vi "PCAN.vi"(8 "error in (no error)":errorcluster, 10 "DUT":string) -> (0 "error in (out)":errorcluster)   [LabVIEW 2024, in "PCANusb_DTU.lvlib"]
doc: "This template is for the Queued Message Handler design pattern.\n\nThe Event Handling Loop generates messages based on user interface actions.\n\nThe Message Handling Loop processes messages generated by the Event Handling Loop, or by other messages. The messages are string values, so new messages can be added easily to the Message Cases case structure in the Message Handling Loop. Each message cluster can also provide an optional value for Message Data, which is a variant that can be converted to whatever message-specific data is required."
uses:
  PCANusb_DTU.lvlib
  support/CAN_MSGs.ctl
  support/CAN_Frames_ctrl.ctl
  support/Framing datas.ctl
  <vilib>/xnet/xnet.llb/XNET Frame CAN.ctl
  <vilib>/xnet/xnet.llb/XNET Frame Type CAN.ctl
  controls/PCAN UI Data.ctl
  support/CAN_Read.ctl
  PrivateControls/FGV_Queue_Control.ctl
  support/PCAN_Global.vi
  Launcher/SubVI/Global 1.vi
  support/Write_frames.vi
  <vilib>/Utility/error.llb/Error Cluster From Error Code.vi
  <vilib>/ErrorRing/Error Ring.xnode
  support/Message Queue/PCAN Message Queue.lvlib
  support/User Event - Stop/PCAN User Event - Stop.lvlib
  <userlib>/PCANBasic/PCANBasic.lvlib
  Launcher/Launcher_DTU.lvlib
  <vilib>/xnet/xnet.llb/XNET Convert (Signal to Frame CAN).vi
panel:
  in  "Config":string
  out "Barcode data":u8[][](array[numeric]) format="%.0x"
  out "CAN_Frames.CAN_ID":u32 format="%.0x"
  out "function return":u32
  out "Channel":u16 format="%.0x"
  out "TPCANMsg":T1[](array[typedef]) {"payload" format="%x"; "timestamp" format="%<%.7X\n%x>T"; "type" items=["CAN Data"=0, "CAN Remote"=1, "CAN Bus Error"=2, "CAN 2.0 Data"=8, "CAN FD Data"=16, "CAN FD+BRS Data"=24, "J1939 Data"=192, "Delay"=224, "Log Trigger"=225, "Start Trigger"=226]; "identifier" format="%x"}
  out "frame data":T1[](array[typedef]) {"payload" format="%x"; "timestamp" format="%<%.7X\n%x>T"; "type" items=["CAN Data"=0, "CAN Remote"=1, "CAN Bus Error"=2, "CAN 2.0 Data"=8, "CAN FD Data"=16, "CAN FD+BRS Data"=24, "J1939 Data"=192, "Delay"=224, "Log Trigger"=225, "Start Trigger"=226]; "identifier" format="%x"}
  out "CAN_bit frame":bool[][](array[boolean])
  in  "CAN_MSGs":T3={"Scaling Factor"=1, "Physical value"=0.0, "CAN_Frames"={"CAN_ID"=0, "MSGTYPE"=128, "Payload"=[], "Length"=0}, "Offset value"=0.0, "Framing datas"=[], "CAN_Frame Enable"=FALSE, "Add Signal"=FALSE, "Delete Signal"=FALSE, "Signal Values"=[], "Time(ms)"=0.0, "Repetition"=FALSE, "Delay"=FALSE, "Delay time"=0.0} {"CAN_Frames"."Payload" format="%.0x"; "CAN_Frames"."MSGTYPE" items=["STATUS"=128, "EXTENDED"=2, "RTR"=1, "DATA MSG"=0]; "CAN_Frames"."CAN_ID" format="%.0x"}
  out "queue name":string
  out "Display <Replace Me>":string
  in  "Read_PCAN":bool
  in  "Write_PCAN":bool
  in  "Exit":bool
  # "Need to build a logic which takes all the bit information,\nbyte info ,Starting bit , Bit length, for each signal with add button to add\nmuch signals manually. And also an option to write payload data for the \nsetup.  - Done."
  # "0     1     2     3     4     5     6     7"
  # "0"
  # "1"
  # "2"
  # "3"
  # "4"
  # "5"
  # "6"
  # "7"
  # "0     1     2     3     4     5     6     7"
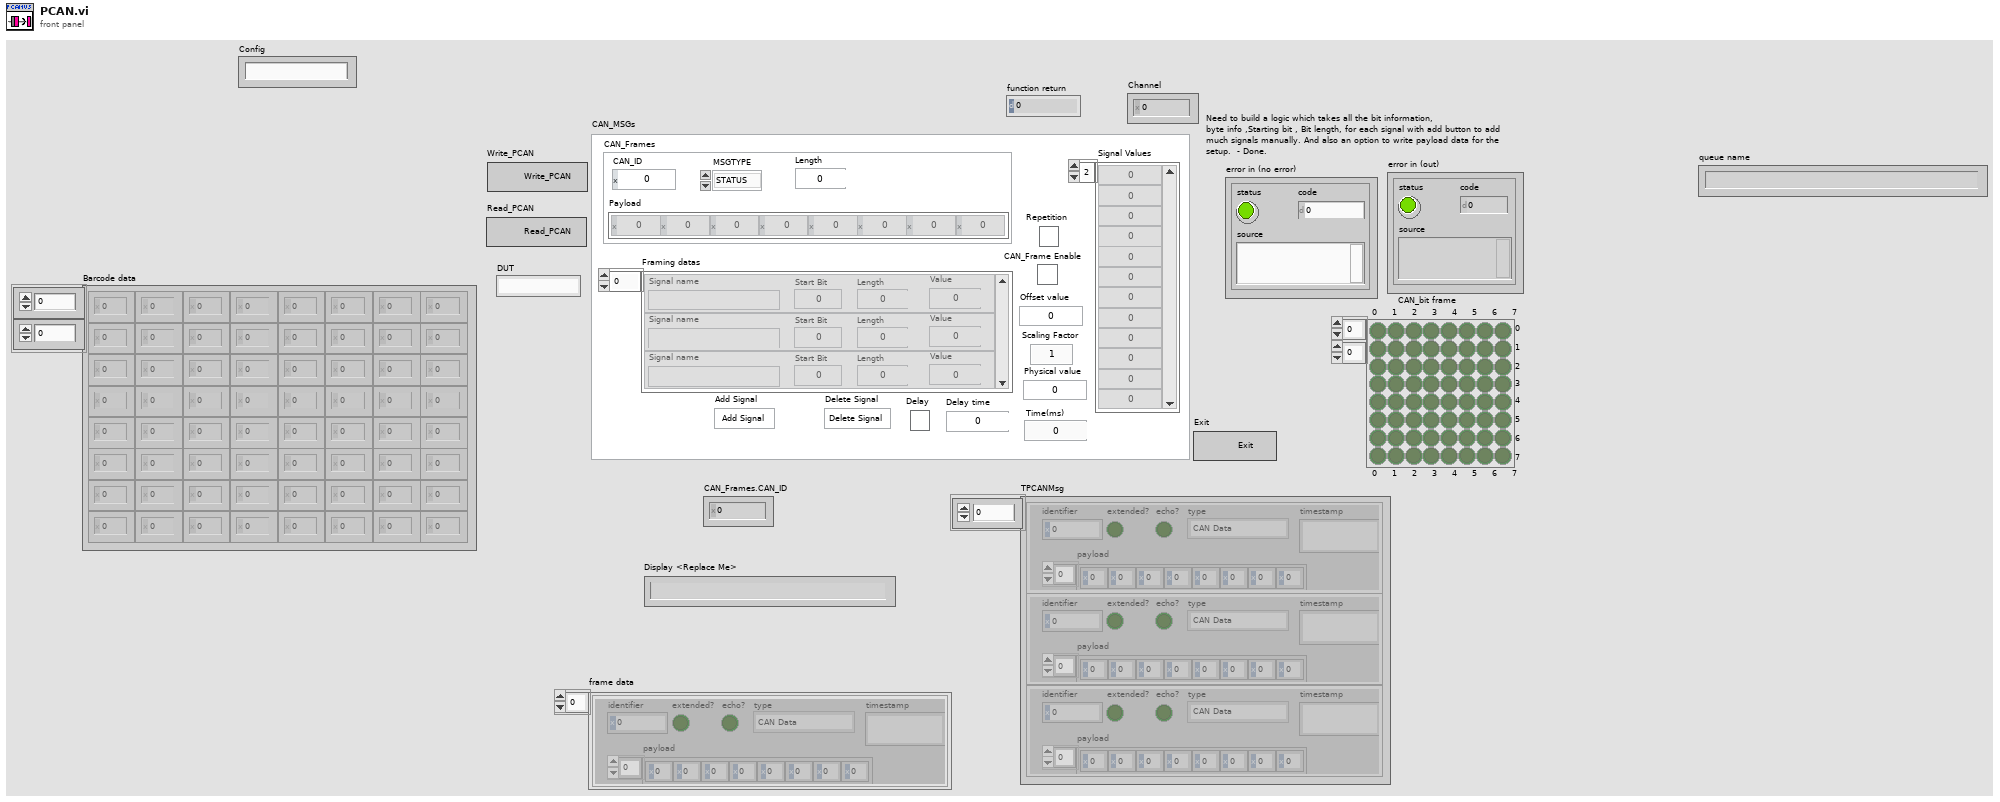
[diagram p1: front panel]
types:
  T1 = typedef "XNET Frame CAN.ctl" = cluster{"timestamp":timestamp, "payload":u8[], "identifier":u32, "type":T2, "extended?":bool, "echo?":bool}
  T2 = typedef "XNET Frame Type CAN.ctl" = u8
  T3 = typedef "PCANusb_DTU.lvlib/CAN_MSGs.ctl" = cluster{"Scaling Factor":u16, "Physical value":dbl, "CAN_Frames":T4, "Offset value":dbl, "Framing datas":T5[], "CAN_Frame Enable":bool, "Add Signal":bool, "Delete Signal":bool, "Signal Values":dbl[], "Time(ms)":dbl, "Repetition":bool, "Delay":bool, "Delay time":dbl}
  T4 = typedef "PCANusb_DTU.lvlib/CAN_Frames_ctrl.ctl" = cluster{"CAN_ID":u32, "MSGTYPE":u8, "Payload":u8[], "Length":u8}
  T5 = typedef "PCANusb_DTU.lvlib/Framing datas.ctl" = cluster{"Signal name":string, "Start Bit":u8, "Length":u8, "Value":u16}
  T6 = cluster{"Message":string, "Message Data":variant}
  T7 = typedef "PCANusb_DTU.lvlib/PCAN UI Data.ctl" = cluster{"DLL_Path":path, "DLL_Path 2":path, "DUT":i32, "CAN_MSGs_Write":T3, "CAN_Array":T3[], "TPCANMsg":cluster{"timestamp":timestamp, "payload":u8[], "identifier":u32, "type":T2, "extended?":bool, "echo?":bool}[], "CAN_Read":T8, "notifier out":refnum<notifier>, "TPCANMsg 2":cluster{"timestamp":timestamp, "payload":u8[], "identifier":u32, "type":T2, "extended?":bool, "echo?":bool}[], "Channel":u16, "reference":refnum<vi>[], "CANand ref":u32[], "CANID Found":bool, "Serial no.":u8[][], "Repeatno.":u8, "GPS":u8[][], "imei":u8[][], "iccid":u8[][], "macid":u8[], "P_queue":refnum<queue>, "Config":string}
  T8 = typedef "PCANusb_DTU.lvlib/CAN_Read.ctl" = cluster{"Database":refnum<k21>, "Signal":refnum<k21>, "BYTES":u32[], "ReadPayload":u8[], "String_Data":string, "ReadValue":dbl, "CANID":u32, "SERVICE ID":u32, "SUB-SERVICE ID":u32, "DELAY ":bool, "Delay time(ms)":dbl}
  T9 = typedef "PCANusb_DTU.lvlib/PCAN Message Queue.lvlib/All Message Queues.ctl" = cluster{"UI":refnum<queue>, "QSM":refnum<queue>}
  T10 = cluster{"timestamp":timestamp, "payload":u8[], "identifier":u32, "type":T2, "extended?":bool, "echo?":bool}[]
  T11 = typedef "PCANusb_DTU.lvlib/FGV_Queue_Control.ctl" = enum16{"Release", "Flush", "Get", "Set"}
  T12 = enum16{"Read", "Write", "All_sections", "All_values", "Remove key&section"}
  T13 = cluster{"millis":u32, "millis_overflow":u16, "micros":u16}
  T14 = cluster{"ID":u32, "MSGTYPE":u8, "LEN":u8, "DATA[0]":u8, "DATA[1]":u8, "DATA[2]":u8, "DATA[3]":u8, "DATA[4]":u8, "DATA[5]":u8, "DATA[6]":u8, "DATA[7]":u8}
  T15 = cluster{"timestamp":timestamp, "payload":u8[], "identifier":u32, "type":T2, "extended?":bool, "echo?":bool}
  T16 = cluster{"ID":u32, "MSGTYPE":u8, "LEN":u8, "aDATA":u8[]}
  T17 = typedef "PCAN_ERROR.ctl" = i32
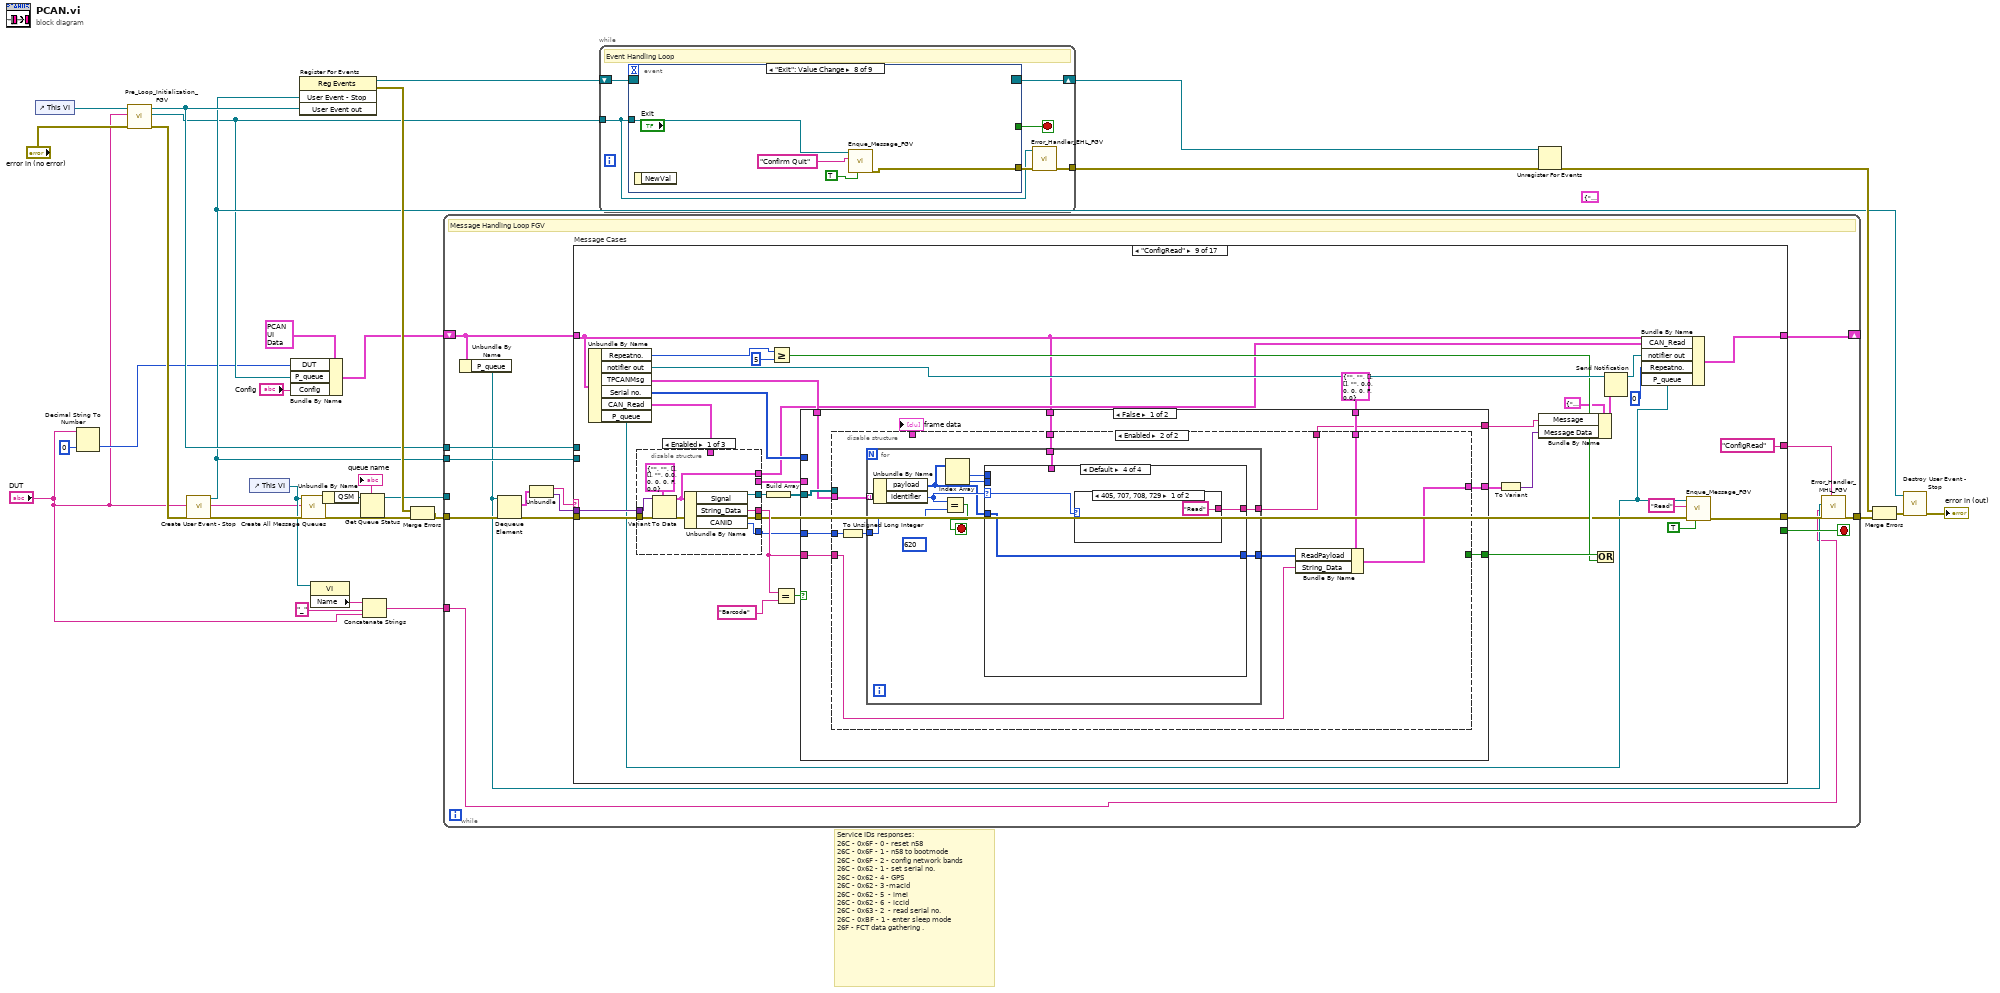
[diagram p0: block diagram]
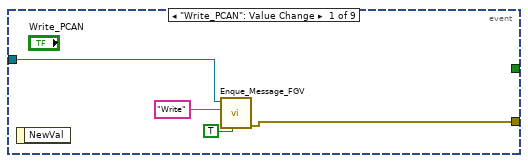
[diagram p2: hidden frame]
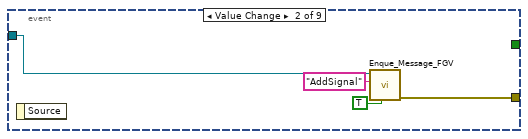
[diagram p3: hidden frame]
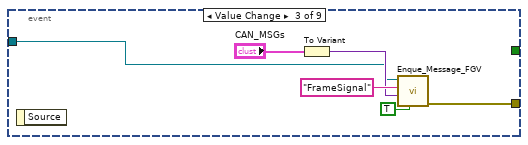
[diagram p4: hidden frame]
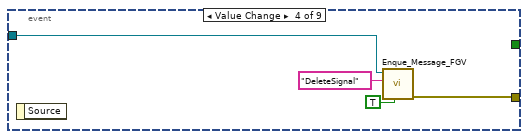
[diagram p5: hidden frame]
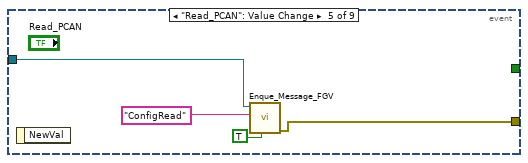
[diagram p6: hidden frame]
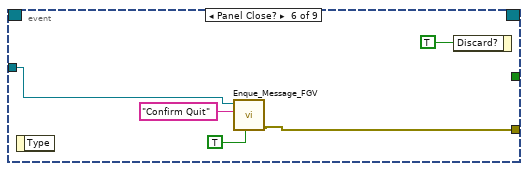
[diagram p7: hidden frame]
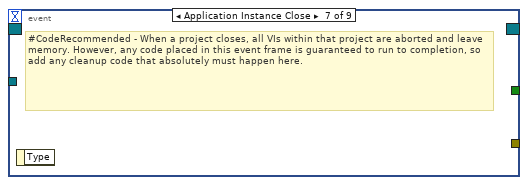
[diagram p8: hidden frame]
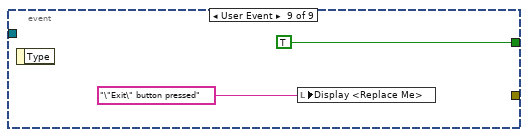
[diagram p9: hidden frame]
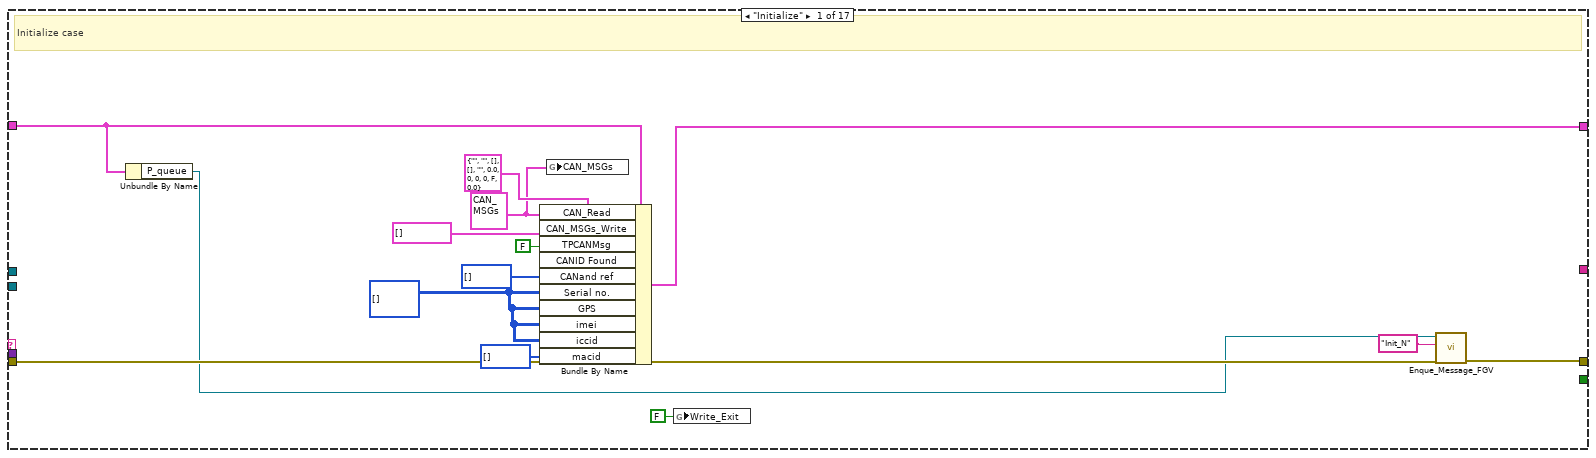
[diagram p10: hidden frame]
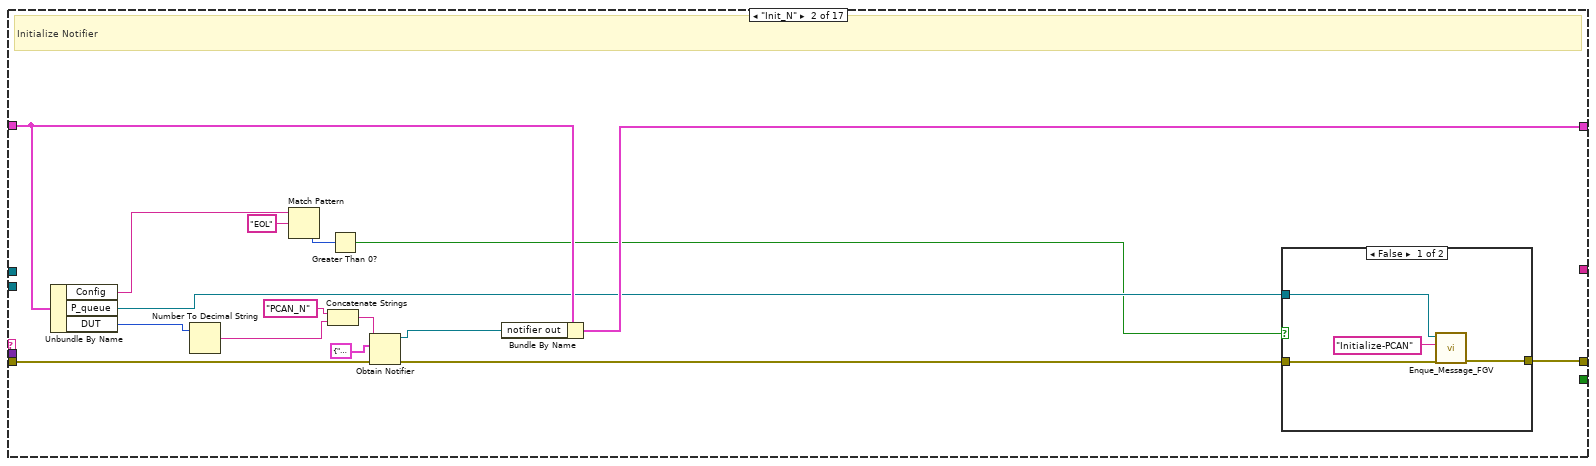
[diagram p11: hidden frame]
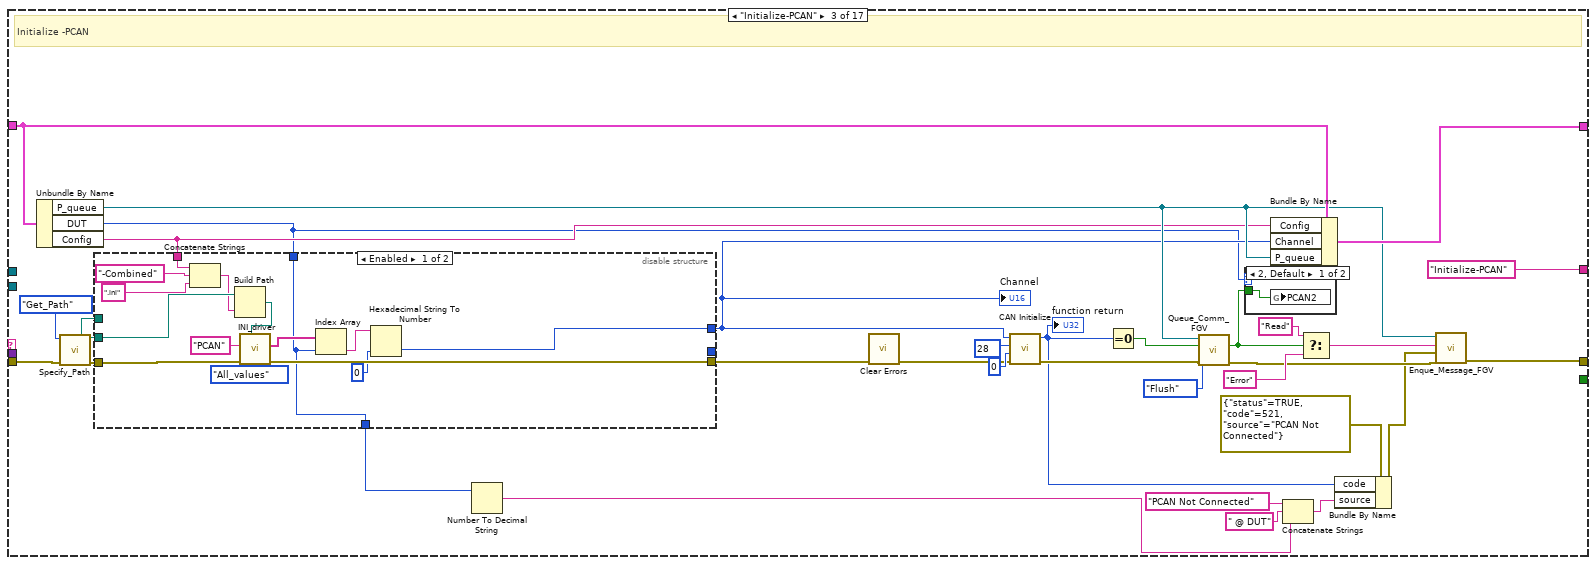
[diagram p13: hidden frame]
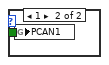
[diagram p14: hidden frame]
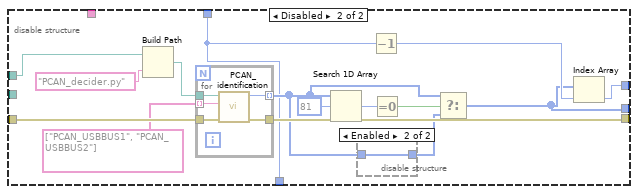
[diagram p15: hidden frame]
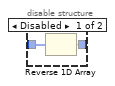
[diagram p16: hidden frame]
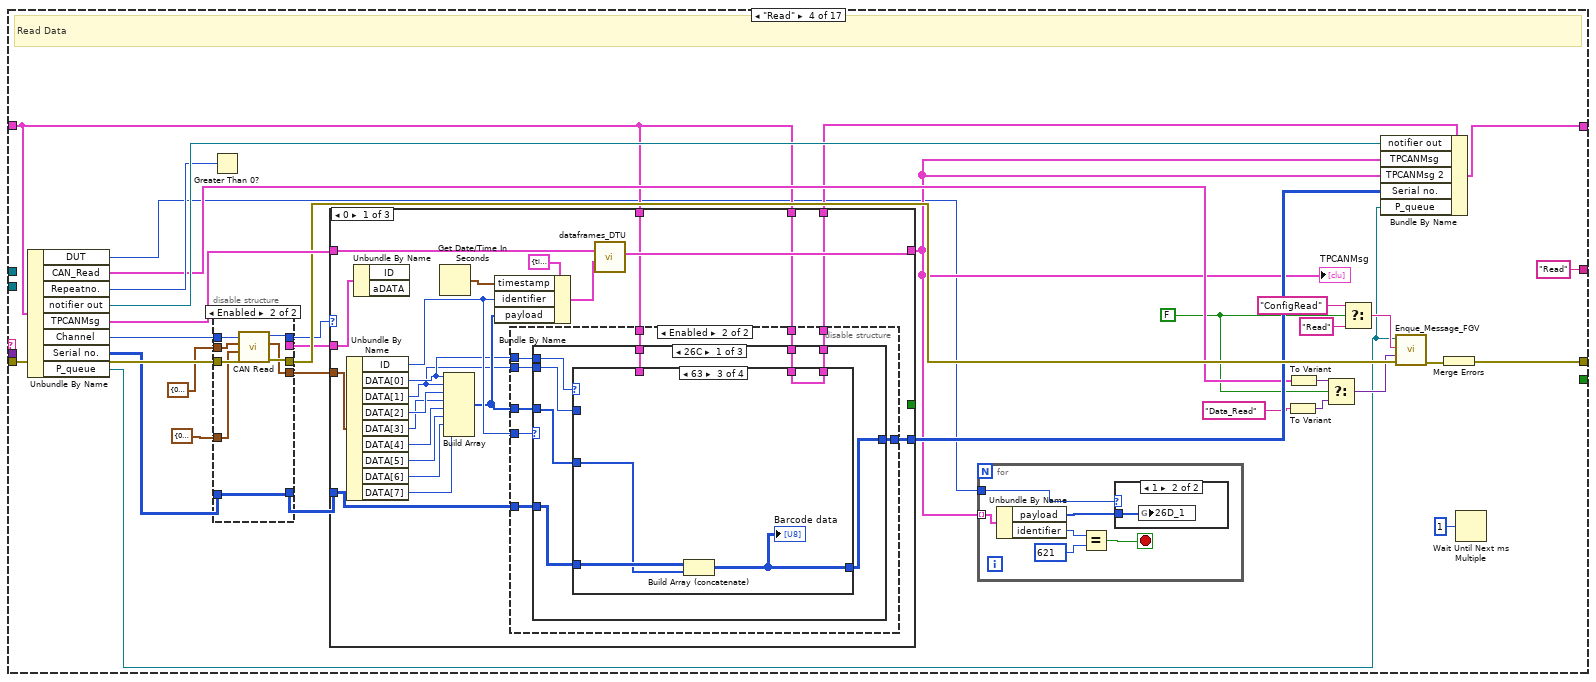
[diagram p17: hidden frame]
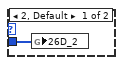
[diagram p18: hidden frame]
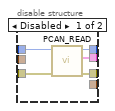
[diagram p19: hidden frame]
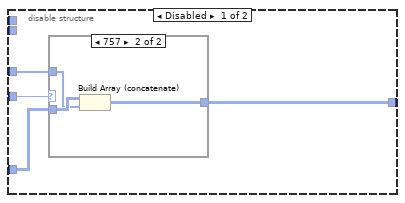
[diagram p20: hidden frame]
diagram:
  (unwired) T6 {"Message"="", "Message Data"=variant} ("notification")
  # "Service IDs responses: \n26C - 0x6F - 0 - reset n58\n26C - 0x6F - 1 - n58 to bootmode\n26C - 0x6F - 2 - config network bands\n26C - 0x62 - 1 - set serial no.\n26C - 0x62 - 4 - GPS\n26C - 0x62 - 3 -macid\n26C - 0x62 - 5  - imei\n26C - 0x62 - 6  - iccid\n26C - 0x63 - 2  - read serial no.\n26C - 0xBF - 1 - enter sleep mode\n26F - FCT data gathering ."
  n1 = control-ref of="This VI"() -> (w19:refnum<vi>)
  n2 = Decimal String To Number(string="DUT", default (0L)=0 ("default (0 I32)")) -> (number=w6:i32)  [unwired: 1 in, 1 out]
  n3 = call "Pre_Loop_Initialization_FGV.vi"("error in (no error)"="error in (no error)", "DUT"="DUT", "VI in"=w19) -> ("error out"=w17:errorcluster, "queue out"=w9:refnum<queue>, "User Event out"=w12:refnum<user-event>)  [unwired: 6 in]
  n4 = call "Create User Event - Stop.vi"("error in (no error)"=w17) -> ("error out"=w13:errorcluster, "User Event - Stop"=w11:refnum<user-event>)  [unwired: 9 in]
  n5 = control-ref of="This VI"() -> (w5:refnum<vi>)
  n6 = Bundle By Name(cluster=T7 {"DLL_Path"=path "", "DLL_Path 2"=path "", "DUT"=1, "CAN_MSGs_Write"={"Scaling Factor"=0, "Physical value"=128.0, "CAN_Frames"={"CAN_ID"=0, "MSGTYPE"=128, "Payload"=[], "Length"=0}, "Offset value"=0.0, "Framing datas"=[], "CAN_Frame Enable"=FALSE, "Add Signal"=FALSE, "Delete Signal"=FALSE, "Signal Values"=[], "Time(ms)"=0.0, "Repetition"=FALSE, "Delay"=FALSE, "Delay time"=0.0}, "CAN_Array"=[], "TPCANMsg"=[{"timestamp"=timestamp(0 s since 1904-01-01), "payload"=[], "identifier"=0, "type"=0, "extended?"=FALSE, "echo?"=FALSE}, {"timestamp"=timestamp(0 s since 1904-01-01), "payload"=[], "identifier"=0, "type"=0, "extended?"=FALSE, "echo?"=FALSE}], "CAN_Read"={"Database"="", "Signal"="", "BYTES"=[], "ReadPayload"=[], "String_Data"="", "ReadValue"=0.0, "CANID"=0, "SERVICE ID"=0, "SUB-SERVICE ID"=0, "DELAY "=FALSE, "Delay time(ms)"=0.0}, "notifier out"=refnum, "TPCANMsg 2"=[{"timestamp"=timestamp(0 s since 1904-01-01), "payload"=[], "identifier"=0, "type"=0, "extended?"=FALSE, "echo?"=FALSE}, {"timestamp"=timestamp(0 s since 1904-01-01), "payload"=[], "identifier"=0, "type"=0, "extended?"=FALSE, "echo?"=FALSE}], "Channel"=81, "reference"=[], "CANand ref"=[], "CANID Found"=FALSE, "Serial no."=[], "Repeatno."=0, "GPS"=[], "imei"=[], "iccid"=[], "macid"=[], "P_queue"=refnum, "Config"=""} ("Data Cluster"), "DUT"=w6, "P_queue"=w9, "Config"="Config") -> (w10:T7)
  n7 = register-events(w11, w12) -> (reference out=w22:refnum<event-registration>, error out=w20:errorcluster)  [unwired: 2 in]
  n8 = call "Create All Message Queues.vi"("error in (no error)"=w13, "DUT"="DUT", "This VI"=w5) -> ("error out"=w31:errorcluster, "Message Queues out"=w30:T9)  [unwired: 7 in]
  n9 = property class="VI"(reference=w5) -> ("Name"=w4:string)  [unwired: 1 in, 2 out]
  n10 = Unbundle By Name(w30) -> ("QSM"=w28:refnum<queue>)
  n11 = Get Queue Status(queue=w28) -> (queue out=w15:refnum<queue>, queue name=→"queue name":string)  [unwired: 2 in, 6 out]
  n12 = Concatenate Strings(w4, "_" ("string"), "DUT") -> (w1:string)
  n13 = Merge Errors(w20, w31) -> (w21:errorcluster)
  n14 = while {
    tunnel: w15 -> [_]
    shift-right: [w46] -> _
    shift-left: w10 -> [w38]
    tunnel: w12 -> [w44]
    tunnel: w21 -> [w43]
    tunnel: [w40] -> w29
    tunnel: w11 -> [w39]
    tunnel: w1 -> [w33]
    stop <- w45 stop-if-true
    # "Message Handling Loop FGV"
    n15 = Unbundle By Name(w38) -> ("P_queue"=w34:refnum<queue>)
    n16 = Dequeue Element(queue=w34, error in (no error)=w43) -> (element=w37:T6, error out=w42:errorcluster)  [unwired: 1 in, 2 out]
    n17 = Unbundle(w37) -> ("Message"=w36:string, "Message Data"=w35:variant)
    n18 = case "Message Cases" shown="\"ConfigRead\"" w36 {
      selector: w36 -> [_ _ _ _ _ _ _ _ _ _ _ _ _ _ _ _ w624]
      tunnel: w42 -> [w58 w75 w102 w184 w314 w364 w374 w387 w424 w558 w567 w577 w582 w590 w599 w609 _]
      tunnel: [w60 w76 w113 w186 w325 w358 w371 w383 w397 w557 w566 w578 w579 w585 w606 w608 w623] -> w41
      tunnel: w38 -> [w48 w73 w97 w160 w329 w356 w367 w382 w396 w556 w565 w572 w583 w584 w602 w614 w625]
      tunnel: [w57 w68 w112 w181 w326 w357 w370 w385 w421 w554 w563 w572 w583 w584 w602 w614 w625] -> w46
      tunnel: [_ _ _ _ _ _ _ _ _ _ _ _ _ _ _ TRUE _] -> w45
      tunnel: w35 -> [_ _ _ _ _ w363 _ w386 w423 _ _ w576 _ w589 _ _ _]
      tunnel: w44 -> [_ _ _ _ _ _ _ _ _ _ _ _ _ _ _ w620 _]
      tunnel: w39 -> [_ _ _ _ _ _ _ _ _ _ _ _ _ _ _ w617 _]
      tunnel: [_ _ "Initialize-PCAN" ("Case") "Read" ("Case") "Write" ("Case") _ _ _ "ConfigRead" ("Case") _ _ _ _ _ _ _ _] -> w32
      frame "Initialize" {
        w50 = u8[][] [] ("Payload")
        w51 = T3 {"Scaling Factor"=1, "Physical value"=0.0, "CAN_Frames"={"CAN_ID"=0, "MSGTYPE"=128, "Payload"=[], "Length"=0}, "Offset value"=0.0, "Framing datas"=[], "CAN_Frame Enable"=FALSE, "Add Signal"=FALSE, "Delete Signal"=FALSE, "Signal Values"=[], "Time(ms)"=0.0, "Repetition"=FALSE, "Delay"=FALSE, "Delay time"=0.0} ("CAN_MSGs_Write")
        # "Initialize case"
        n19 = Unbundle By Name(w48) -> ("P_queue"=w47:refnum<queue>)
        n20 = Bundle By Name(cluster=w48, "CAN_Read"=T8 {"Database"="", "Signal"="", "BYTES"=[], "ReadPayload"=[], "String_Data"="", "ReadValue"=0.0, "CANID"=0, "SERVICE ID"=0, "SUB-SERVICE ID"=0, "DELAY "=FALSE, "Delay time(ms)"=0.0}, "CAN_MSGs_Write"=w51, "TPCANMsg"=T10 [], "CANID Found"=FALSE, "CANand ref"=u32[] [], "Serial no."=w50, "GPS"=w50, "imei"=w50, "iccid"=w50, "macid"=u8[] []) -> (w57:T7)
        n21 = global write "PCAN_Global.vi" "CAN_MSGs"(w51) -> ()
        n22 = global write "PCAN_Global.vi" "Write_Exit"(FALSE ("Write_Exit")) -> ()
        n23 = call "Enque_Message_FGV.vi"("error in (no error)"=w58, "Message"="Init_N", "queue IN"=w47) -> ("error out"=w60:errorcluster)  [unwired: 8 in]
      }
      frame "Init_N" {
        # "Initialize Notifier"
        n24 = Unbundle By Name(w73) -> ("Config"=w62:string, "P_queue"=w66:refnum<queue>, "DUT"=w72:i32)
        n25 = Number To Decimal String(number=w72) -> (decimal integer string=w65:string)  [unwired: 1 in]
        n26 = Match Pattern(string=w62, regular expression="EOL") -> (offset past match=w63:i32)  [unwired: 1 in, 3 out]
        n27 = Concatenate Strings("PCAN_N" ("String"), w65) -> (w71:string)
        n28 = Greater Than 0?(x=w63) -> (x > 0?=w61:bool)
        n29 = Obtain Notifier(name (unnamed)=w71, notification data type=T6 {"Message"="", "Message Data"=variant} ("notification"), error in (no error)=w75) -> (notifier out=w67:refnum<notifier>, error out=w74:errorcluster)  [unwired: 1 in, 1 out]
        n30 = Bundle By Name(cluster=w73, "notifier out"=w67) -> (w68:T7)
        n31 = case shown="False" w61 {
          tunnel: [w80 w81] -> w76
          tunnel: w74 -> [w78 w81]
          tunnel: w66 -> [w77 _]
          frame False {
            n32 = call "Enque_Message_FGV.vi"("error in (no error)"=w78, "Message"="Initialize-PCAN", "queue IN"=w77) -> ("error out"=w80:errorcluster)  [unwired: 8 in]
          }
          frame True {
          }
        }
      }
      frame "Initialize-PCAN" {
        # "Initialize -PCAN"
        n33 = Unbundle By Name(w97) -> ("P_queue"=w96:refnum<queue>, "DUT"=w82:i32, "Config"=w95:string)
        n34 = call "Specify_Path.vi"("Path_Enum"=enum16{"Find_Path", "Get_Path"}."Get_Path", "error in (no error)"=w102) -> ("stripped path"=w93:path, "Configurations"=w98:path, "error out"=w101:errorcluster)  [unwired: 6 in, 5 out]
        n35 = disable-structure shown="Enabled" {
          disable-tunnel: w101 -> [w130 w145]
          disable-tunnel: [w129 w140] -> w99
          disable-tunnel: w98 -> [w127 _]
          disable-tunnel: w82 -> [w116 w131]
          disable-tunnel: w95 -> [w118 _]
          disable-tunnel: w93 -> [_ w142]
          disable-tunnel: [w117 w135] -> w89
          disable-tunnel: [_ w132] -> _
          disable-tunnel: [w116 w131] -> w85
          frame Enabled {
            n36 = Concatenate Strings(w118, "-Combined" ("string"), ".ini" ("string")) -> (w119:string)
            n37 = Build Path(base path=w127, name or relative path=w119) -> (appended path=w128:path)
            n38 = call "INI_driver.vi"("Enum"=T12."All_values", "instrument file path"=w128, "error in (no error)"=w130, "Section"="PCAN") -> ("error out"=w129:errorcluster, "Values out"=w124:string[])  [unwired: 4 in, 2 out]
            n39 = Index Array(array=w124, index=w116) -> (element=w123:string)
            n40 = Hexadecimal String To Number(string=w123, default (0uL)=u16 0 ("default (0 U32)")) -> (number=w117:u16)  [unwired: 1 in, 1 out]
          }
          frame Disabled {
            n41 = Build Path(base path=w142, name or relative path="PCAN_decider.py") -> (appended path=w144:path)
            n42 = for {
              tunnel: w145 -> [w153]
              tunnel: w144 -> [w152]
              tunnel: string[] ["PCAN_USBBUS1", "PCAN_USBBUS2"] ("PCAN_ID") -> [w151] mode=indexing
              tunnel: [w150] -> w140
              tunnel: [w149] -> w134 mode=indexing
              n43 = call "PCAN_identification.vi"("error in (no error)"=w153, "PCAN_ID"=w151, "module path"=w152) -> ("error out"=w150:errorcluster, "return value"=w149:i32)  [unwired: 7 in]
            }
            n44 = Search 1D Array(1D array=w134, element=81) -> (index of element=w137:i32)  [unwired: 1 in]
            n45 = disable-structure shown="Enabled" {
              disable-tunnel: w134 -> [w147 w148]
              disable-tunnel: [w146 w148] -> w133
              frame Disabled {
                n46 = Reverse 1D Array(array=w147) -> (reversed array=w146:i32[])
              }
              frame Enabled {
              }
            }
            n47 = Decrement(x=w131) -> (x-1=w139:i32)
            n48 = Equal To 0?(x=w137) -> (x = 0?=w136:bool)
            n49 = Select(t=w134, s=w136, f=w133) -> (s? t:f=w132:i32[])
            n50 = Index Array(array=w132, index=w139) -> (element=w135:i32)
          }
        }
        "Channel" <- w89
        n51 = Number To Decimal String(number=w85) -> (decimal integer string=w84:string)  [unwired: 1 in]
        n52 = call <vilib>:"Clear Errors.vi"("error in (no error)"=w99) -> ("error out"=w92:errorcluster)  [unwired: 5 in, 1 out]
        n53 = call <userlib>:"CAN Initialize.vi"("error in (no error)"=w92, "HwType"=u8 0, "Btr0Btr1"=u16 28, "Channel"=w89) -> ("error out"=w103:errorcluster, "function return"=w90:u32)  [unwired: 6 in]
        "function return" <- w90
        n54 = Equal To 0?(x=w90) -> (x = 0?=w83:bool)
        n55 = call "Queue_Comm_FGV.vi"("error in (no error)"=w103, "Enum"=FGV_Queue_Control."Flush", "queue in"=w96) -> ("error Out"=w105:errorcluster)  [unwired: 7 in, 1 out]
        n56 = case shown="2, Default" w82 {
          tunnel: w83 -> [w114 w115]
          frame 2, Default {
            n57 = global write "Global 1.vi" "PCAN2"(w114) -> ()
          }
          frame 1 {
            n58 = global write "Global 1.vi" "PCAN1"(w115) -> ()
          }
        }
        n59 = Bundle By Name(cluster=w97, "Config"=w95, "Channel"=w89, "P_queue"=w96) -> (w112:T7)
        n60 = Concatenate Strings("PCAN Not Connected" ("source"), " @ DUT" ("string"), w84) -> (w88:string)
        n61 = Select(t="Read" ("Message"), s=w83, f="Error" ("Message")) -> (s? t:f=w109:string)
        n62 = Bundle By Name(cluster=errorcluster {"status"=TRUE, "code"=521, "source"="PCAN Not Connected"} ("error constant"), "code"=w90, "source"=w88) -> (w91:errorcluster)
        n63 = call "Enque_Message_FGV.vi"("error in (no error)"=w105, "Message Data"=w91, "Message"=w109, "queue IN"=w96) -> ("error out"=w113:errorcluster)  [unwired: 7 in]
      }
      frame "Read" {
        w161 = FALSE
        # "Read Data"
        n64 = Unbundle By Name(w160) -> ("DUT"=w156:i32, "CAN_Read"=w162:T8, "Repeatno."=w170:u8, "notifier out"=w180:refnum<notifier>, "TPCANMsg"=w183:T10, "Channel"=w154:u16, "Serial no."=w172:u8[][], "P_queue"=w158:refnum<queue>)
        n65 = Greater Than 0?(x=w170) -> ()  [unwired: 1 out]
        n66 = disable-structure shown="Enabled" {
          disable-tunnel: w184 -> [w199 w206]
          disable-tunnel: w154 -> [w198 w201]
          disable-tunnel: [w197 w207] -> w182
          disable-tunnel: [w196 w205] -> w178
          disable-tunnel: [w195 _] -> w177
          disable-tunnel: T14 {"ID"=0, "MSGTYPE"=0, "LEN"=0, "DATA[0]"=0, "DATA[1]"=0, "DATA[2]"=0, "DATA[3]"=0, "DATA[4]"=0, "DATA[5]"=0, "DATA[6]"=0, "DATA[7]"=0} ("MessageBuffer") -> [_ w204]
          disable-tunnel: T13 {"millis"=0, "millis_overflow"=0, "micros"=0} ("TimestampBuffer") -> [_ w203]
          disable-tunnel: [_ w202] -> w174
          disable-tunnel: [_ w200] -> w173
          disable-tunnel: w172 -> [_ w200]
          frame Disabled {
            n67 = call <vilib>:"PCAN_READ.vi"("error in (no error)"=w199, "path in"=w198) -> ("error out"=w197:errorcluster, "TPCANMsg"=w195:T16, "error"=w196:T17)  [unwired: 6 in, 1 out]
          }
          frame Enabled {
            n68 = call <userlib>:"CAN Read.vi"("error in (no error)"=w206, "TimestampBuffer"=w203, "MessageBuffer"=w204, "Channel"=w201) -> ("error out"=w207:errorcluster, "MessageBuffer out"=w202:T14, "function return"=w205:u32)  [unwired: 4 in, 1 out]
          }
        }
        n69 = case shown="0" w178 {
          tunnel: [_ TRUE TRUE] -> _
          tunnel: w177 -> [w229 _ _]
          tunnel: w183 -> [w226 w298 w302]
          tunnel: [w225 w298 w302] -> w157
          tunnel: w174 -> [w223 _ _]
          tunnel: w173 -> [w215 w297 w301]
          tunnel: [w213 w297 w301] -> w171
          tunnel: w160 -> [w210 _ _]
          tunnel: w160 -> [w209 w296 w300]
          tunnel: [w208 w296 w300] -> w159
          frame 0 {
            n70 = Unbundle By Name(w223) -> ("ID"=w216:u32, "DATA[0]"=w212:u8, "DATA[1]"=w211:u8, "DATA[2]"=w222:u8, "DATA[3]"=w221:u8, "DATA[4]"=w220:u8, "DATA[5]"=w219:u8, "DATA[6]"=w218:u8, "DATA[7]"=w217:u8)
            n71 = Unbundle By Name(w229) -> ()  [unwired: 2 out]
            n72 = Get Date/Time In Seconds() -> (seconds since 1Jan1904=w227:timestamp)
            n73 = Build Array(w212, w211, w222, w221, w220, w219, w218, w217) -> (w214:u8[])
            n74 = Bundle By Name(cluster=T15 {"timestamp"=timestamp(0 s since 1904-01-01), "payload"=[], "identifier"=0, "type"=0, "extended?"=FALSE, "echo?"=FALSE} ("CAN frame"), "timestamp"=w227, "identifier"=w216, "payload"=w214) -> (w224:T15)
            n75 = disable-structure shown="Enabled" {
              disable-tunnel: w216 -> [w233 w246]
              disable-tunnel: w215 -> [w232 w245]
              disable-tunnel: w214 -> [w231 w238]
              disable-tunnel: [w230 w244] -> w213
              disable-tunnel: w212 -> [_ w243]
              disable-tunnel: w211 -> [_ w242]
              disable-tunnel: w210 -> [_ w241]
              disable-tunnel: w209 -> [_ w240]
              disable-tunnel: [_ w239] -> w208
              frame Disabled {
                n76 = case shown="757" w233 {
                  tunnel: w232 -> [w234 w237]
                  tunnel: w231 -> [_ w236]
                  tunnel: [w234 w235] -> w230
                  frame 0, Default {
                  }
                  frame 1879 {
                    n77 = Build Array (concatenate)(w237, w236) -> (w235:u8[][])
                  }
                }
              }
              frame Enabled {
                n78 = case shown="26C" w246 {
                  tunnel: w245 -> [w248 w293 w295]
                  tunnel: [w247 w293 w295] -> w244
                  tunnel: w243 -> [w254 _ _]
                  tunnel: w242 -> [w253 _ _]
                  tunnel: w241 -> [w252 _ _]
                  tunnel: w240 -> [w251 w292 w294]
                  tunnel: [w250 w292 w294] -> w239
                  tunnel: w238 -> [w249 _ _]
                  frame 620 {
                    n79 = case shown="63" w254 {
                      tunnel: w253 -> [w257 w263 _ _]
                      tunnel: w252 -> [_ w262 _ _]
                      tunnel: w251 -> [w255 w261 w289 w290]
                      tunnel: [w255 w260 w289 w290] -> w250
                      tunnel: w249 -> [_ w259 w287 _]
                      tunnel: w248 -> [w256 w258 w288 w291]
                      tunnel: [w256 w258 w286 w291] -> w247
                      frame 111, Default {
                        n80 = case shown="0, Default" w257 {
                          frame 0, Default {
                          }
                          frame 1 {
                          }
                        }
                      }
                      frame 98 {
                        n81 = case shown="3" w263 {
                          tunnel: w262 -> [_ w270 _ w279 w285]
                          tunnel: w261 -> [w264 w269 w273 w278 w284]
                          tunnel: [w264 w268 w272 w277 w283] -> w260
                          tunnel: w259 -> [_ w266 w271 w274 w280]
                          frame 1, Default {
                          }
                          frame 4 {
                            # "GPS"
                            n82 = Unbundle By Name(w270) -> ("GPS"=w267:u8[][])
                            n83 = Build Array (concatenate)(w267, w266) -> (w265:u8[][])
                            n84 = Bundle By Name(cluster=w269, "GPS"=w265) -> (w268:T7)
                          }
                          frame 3 {
                            n85 = Bundle By Name(cluster=w273, "macid"=w271) -> (w272:T7)
                          }
                          frame 5 {
                            n86 = Unbundle By Name(w279) -> ("imei"=w276:u8[][])
                            n87 = Build Array (concatenate)(w276, w274) -> (w275:u8[][])
                            n88 = Bundle By Name(cluster=w278, "imei"=w275) -> (w277:T7)
                          }
                          frame 6 {
                            n89 = Unbundle By Name(w285) -> ("iccid"=w282:u8[][])
                            n90 = Build Array (concatenate)(w282, w280) -> (w281:u8[][])
                            n91 = Bundle By Name(cluster=w284, "iccid"=w281) -> (w283:T7)
                          }
                        }
                      }
                      frame 99 {
                        n92 = Build Array (concatenate)(w288, w287) -> (w286:u8[][])
                        "Barcode data" <- w286
                      }
                      frame 191 {
                      }
                    }
                  }
                  frame 623 {
                  }
                  frame Default {
                  }
                }
              }
            }
            n93 = call "dataframes_DTU.vi"("input cluster"=w224, "frame data"=w226) -> ("frame data 2"=w225:T1[])  [unwired: 9 in]
          }
          frame 32 {
          }
          frame Default {
          }
        }
        "TPCANMsg" <- w157
        n94 = for {
          tunnel: w157 -> [w192] mode=indexing
          tunnel: w156 -> [w188]
          stop <- w189 stop-if-true
          n95 = Unbundle By Name(w192) -> ("payload"=w187:u8[], "identifier"=w190:u32)
          n96 = Equal?(x=w190, y=u32 621 ("identifier")) -> (x = y?=w189:bool)
          n97 = case shown="1" w188 {
            tunnel: w187 -> [w193 w194]
            frame 2, Default {
              n98 = global write "PCAN_Global.vi" "26D_2"(w193) -> ()
            }
            frame 1 {
              n99 = global write "PCAN_Global.vi" "26D_1"(w194) -> ()
            }
          }
        }
        n100 = To Variant(anything="Data_Read" ("\"Do Something\" button pressed")) -> (Variant=w164:variant)
        n101 = To Variant(anything=w162) -> (Variant=w166:variant)
        n102 = Select(t=w166, s=w161, f=w164) -> (s? t:f=w163:variant)
        n103 = Select(t="ConfigRead", s=w161, f="Read" ("Message")) -> (s? t:f=w167:string)
        n104 = Bundle By Name(cluster=w159, "notifier out"=w180, "TPCANMsg"=w157, "TPCANMsg 2"=w157, "Serial no."=w171, "P_queue"=w158) -> (w181:T7)
        n105 = call "Enque_Message_FGV.vi"("error in (no error)"=w182, "Message Data"=w163, "Message"=w167, "queue IN"=w158) -> ("error out"=w185:errorcluster)  [unwired: 7 in]
        n106 = Merge Errors(w185) -> (w186:errorcluster)
        n107 = Wait Until Next ms Multiple(millisecond multiple=u32 1) -> ()  [unwired: 1 out]
      }
      frame "Write" {
        w308 = u8[][] [] ("Payload")
        # "CAN Write"
        n108 = Unbundle By Name(w329) -> ("notifier out"=w327:refnum<notifier>, "Channel"=w312:u16, "CAN_MSGs_Write"=w311:T3, "CANand ref"=w310:u32[], "P_queue"=w307:refnum<queue>)  [unwired: 1 out]
        n109 = case shown="False" FALSE {
          tunnel: w314 -> [w346 w349]
          tunnel: [w345 w349] -> w313
          tunnel: w312 -> [w341 _]
          tunnel: w311 -> [w335 w347]
          tunnel: w310 -> [w334 w348]
          tunnel: [w332 w348] -> w309
          frame False {
            n110 = Unbundle By Name(w335) -> ("CAN_Frames.CAN_ID"=w333:u32)
            "CAN_Frames.CAN_ID" <- w333
            n111 = To Variant(anything=w335) -> (Variant=w340:variant)
            n112 = To Variant(anything=w341) -> (Variant=w339:variant)
            n113 = vi-ref "PCANusb_DTU.lvlib:Write_frames.vi"() -> (w343:refnum<vi>)
            n114 = Build Array(w340, w339) -> (w338:variant[])
            n115 = Build Array (concatenate)(w334, w333) -> (w332:u32[])
            n116 = call "Dynamic launcher.vi"("element"=string[] ["CAN_MSGs_Write", "Channel"], "Clone ?"=TRUE, "Value"=w338, "VI Refnum"=w343, "error in (no error)"=w346, "Open FP"=FALSE, "options"=8) -> ("error out"=w345:errorcluster)  [unwired: 6 in, 2 out]
          }
          frame True {
            n117 = global write "PCAN_Global.vi" "CAN_MSGs"(w347) -> ()
          }
        }
        n118 = Unbundle By Name(w313) -> ("status"=w318:bool)
        n119 = call <vilib>:"Clear Errors.vi"("error in (no error)"=w313) -> ("error out"=w323:errorcluster)  [unwired: 5 in, 1 out]
        n120 = Not(x=w318) -> (.not. x?=w317:bool)
        n121 = Select(t="Step_Done" ("Message"), s=w317, f="Error") -> (s? t:f=w319:string)
        n122 = Bundle By Name(cluster=T6 {"Message"="", "Message Data"=variant} ("notification"), "Message"=w319) -> (w320:T6)
        n123 = Send Notification(notification=w320, notifier=w327, error in (no error)=w323) -> (notifier out=w315:refnum<notifier>, error out=w324:errorcluster)
        n124 = call "Enque_Message_FGV.vi"("Priority"=TRUE, "error in (no error)"=w313, "Message Data"="Write CAN " ("\"Do Something Else\" button pressed"), "Message"="Read", "queue IN"=w307) -> ("error out"=w328:errorcluster)  [unwired: 6 in]
        n125 = Bundle By Name(cluster=w329, "Serial no."=w308, "notifier out"=w315, "CANand ref"=w309, "GPS"=w308, "imei"=w308, "iccid"=w308, "P_queue"=w307) -> (w326:T7)
        n126 = Merge Errors(w324, w328) -> (w325:errorcluster)
      }
      frame "FrameSignal" {
        # "Frame Signal"
        n127 = Unbundle By Name(w356) -> ("CANand ref"=w354:u32[], "P_queue"=w350:refnum<queue>)
        n128 = Variant To Data(error in=w364, type=T3 {"Scaling Factor"=1, "Physical value"=0.0, "CAN_Frames"={"CAN_ID"=0, "MSGTYPE"=128, "Payload"=[], "Length"=0}, "Offset value"=0.0, "Framing datas"=[], "CAN_Frame Enable"=FALSE, "Add Signal"=FALSE, "Delete Signal"=FALSE, "Signal Values"=[], "Time(ms)"=0.0, "Repetition"=FALSE, "Delay"=FALSE, "Delay time"=0.0} ("CAN_MSGs"), Variant=w363) -> (data=w355:T3, error out=w359:errorcluster)
        n129 = Unbundle By Name(w355) -> ("CAN_Frames.CAN_ID"=w353:u32)
        n130 = Search 1D Array(1D array=w354, element=w353) -> (index of element=w352:i32)  [unwired: 1 in]
        n131 = Less Than 0?(x=w352) -> (x < 0?=w351:bool)
        n132 = Bundle By Name(cluster=w356, "CANID Found"=w351, "CAN_MSGs_Write"=w355) -> (w357:T7)
        n133 = call "Enque_Message_FGV.vi"("error in (no error)"=w359, "Message Data"="Frame Signal" ("\"Do Something Else\" button pressed"), "Message"="Update Display", "queue IN"=w350) -> ("error out"=w358:errorcluster)  [unwired: 7 in]
      }
      frame "Reset" {
        # "ResetIDs"
        n134 = Unbundle By Name(w367) -> ("P_queue"=w366:refnum<queue>)
        n135 = Bundle By Name(cluster=w367, "CANand ref"=u32[] [], "CANID Found"=FALSE, "TPCANMsg"=T10 []) -> (w370:T7)
        n136 = call "Enque_Message_FGV.vi"("error in (no error)"=w374, "Message Data"="ResetIDs" ("\"Do Something Else\" button pressed"), "Message"="Read", "queue IN"=w366) -> ("error out"=w371:errorcluster)  [unwired: 7 in]
      }
      frame "ConfigWrite" {
        n137 = Unbundle By Name(w382) -> ("P_queue"=w375:refnum<queue>, "CANand ref"=w380:u32[])
        n138 = Variant To Data(error in=w387, type=T3 {"Scaling Factor"=1, "Physical value"=0.0, "CAN_Frames"={"CAN_ID"=0, "MSGTYPE"=128, "Payload"=[], "Length"=0}, "Offset value"=0.0, "Framing datas"=[], "CAN_Frame Enable"=FALSE, "Add Signal"=FALSE, "Delete Signal"=FALSE, "Signal Values"=[], "Time(ms)"=0.0, "Repetition"=FALSE, "Delay"=FALSE, "Delay time"=0.0} ("CAN_MSGs"), Variant=w386) -> (data=w381:T3, error out=w384:errorcluster)
        n139 = Unbundle By Name(w381) -> ("CAN_Frames.CAN_ID"=w379:u32)
        n140 = Search 1D Array(1D array=w380, element=w379) -> (index of element=w378:i32)  [unwired: 1 in]
        n141 = Less Than 0?(x=w378) -> ()  [unwired: 1 out]
        n142 = Bundle By Name(cluster=w382, "CANID Found"=FALSE, "CAN_MSGs_Write"=w381) -> (w385:T7)
        n143 = call "Enque_Message_FGV.vi"("Priority"=TRUE, "error in (no error)"=w384, "Message Data"="Config Write" ("\"Do Something Else\" button pressed"), "Message"="Write", "queue IN"=w375) -> ("error out"=w383:errorcluster)  [unwired: 6 in]
      }
      frame "ConfigRead" {
        n144 = Unbundle By Name(w396) -> ("Repeatno."=w401:u8, "notifier out"=w422:refnum<notifier>, "TPCANMsg"=w418:T10, "Serial no."=w413:u8[][], "CAN_Read"=w412:T8, "P_queue"=w394:refnum<queue>)
        n145 = disable-structure shown="Enabled" {
          disable-tunnel: w424 -> [w542 w546 w551]
          disable-tunnel: [w541 w545 w551] -> w398
          disable-tunnel: w423 -> [w540 w544 _]
          disable-tunnel: [w538 _ w549] -> w420
          disable-tunnel: [w537 _ w548] -> w415
          disable-tunnel: w412 -> [_ _ w550]
          disable-tunnel: [w536 _ _] -> w411
          disable-tunnel: [w535 w543 _] -> w402
          disable-tunnel: [_ w543 _] -> w400
          frame Enabled {
            n146 = Variant To Data(error in=w542, type=T8 {"Database"="", "Signal"="", "BYTES"=[], "ReadPayload"=[], "String_Data"="", "ReadValue"=0.0, "CANID"=0, "SERVICE ID"=0, "SUB-SERVICE ID"=0, "DELAY "=FALSE, "Delay time(ms)"=0.0} ("CAN_Read"), Variant=w540) -> (data=w535:T8, error out=w541:errorcluster)
            n147 = Unbundle By Name(w535) -> ("Signal"=w538:refnum<k21>, "String_Data"=w537:string, "CANID"=w536:u32)
          }
          frame Disabled {
            n148 = Variant To Data(error in=w546, type=T8 {"Database"="", "Signal"="", "BYTES"=[], "ReadPayload"=[], "String_Data"="", "ReadValue"=0.0, "CANID"=0, "SERVICE ID"=0, "SUB-SERVICE ID"=0, "DELAY "=FALSE, "Delay time(ms)"=0.0} ("CAN_Read"), Variant=w544) -> (data=w543:T8, error out=w545:errorcluster)
          }
          frame Disabled {
            n149 = Unbundle By Name(w550) -> ("Signal"=w549:refnum<k21>, "String_Data"=w548:string)
          }
        }
        n150 = Build Array(w420) -> (w419:refnum<k21>[])
        n151 = Greater Or Equal?(x=w401, y=u8 5) -> (x >= y?=w408:bool)
        n152 = Equal?(x=w415, y="Barcode") -> (x = y?=w416:bool)
        n153 = case shown="False" w416 {
          tunnel: w419 -> [w434 _]
          tunnel: w418 -> [w433 _]
          tunnel: T8 {"Database"="", "Signal"="", "BYTES"=[], "ReadPayload"=[], "String_Data"="", "ReadValue"=0.0, "CANID"=0, "SERVICE ID"=0, "SUB-SERVICE ID"=0, "DELAY "=FALSE, "Delay time(ms)"=0.0} ("CAN_Read") -> [w432 w533]
          tunnel: [w431 w534] -> w395
          tunnel: w415 -> [w430 w532]
          tunnel: w413 -> [_ w531]
          tunnel: w411 -> [w429 _]
          tunnel: [w428 TRUE] -> w410
          tunnel: w400 -> [_ _]
          tunnel: w396 -> [w426 _]
          tunnel: [w425 "Read"] -> w391
          frame False {
            n154 = disable-structure shown="Enabled" {
              disable-tunnel: w434 -> [w448 _]
              disable-tunnel: w433 -> [w447 w457]
              disable-tunnel: w432 -> [w444 w453]
              disable-tunnel: [w442 w451] -> w431
              disable-tunnel: w430 -> [w440 w450]
              disable-tunnel: w429 -> [w437 w456]
              disable-tunnel: [w436 _] -> w428
              disable-tunnel: [w435 _] -> w427
              disable-tunnel: w426 -> [_ w454]
              disable-tunnel: [_ w449] -> w425
              frame Disabled {
                n155 = call <vilib>:"PCAN_CAN_Raw_Frames.vi"("frame data"=w447, "signal list"=w448) -> ("signal data"=w441:dbl[], "session out"=w446:refnum<k21>)  [unwired: 6 in, 2 out]
                n156 = call-poly <vilib>:"XNET Convert.vi"("session in"=w446, "signal data"=w441) -> ("frame data"=w435:T1[])  [unwired: 10 in, 3 out]
                n157 = Index Array(array=w441) -> (element=w439:dbl)  [unwired: 1 in]
                n158 = Index Array(array=w435) -> (element=w445:T1)  [unwired: 1 in]
                n159 = Unbundle By Name(w445) -> ("payload"=w443:u8[])
                n160 = Absolute Value(x=w439) -> (abs(x)=w438:dbl)
                n161 = Bundle By Name(cluster=w444, "ReadPayload"=w443, "String_Data"=w440, "ReadValue"=w438) -> (w442:T8)
                n162 = Equal?(x=w438, y=w437) -> (x = y?=w436:bool)
              }
              frame Enabled {
                n163 = To Unsigned Long Integer(number=w456) -> (unsigned 32bit integer=w455:u32)
                n164 = for {
                  tunnel: w457 -> [w467] mode=indexing
                  tunnel: [w459] -> w452
                  tunnel: w455 -> [w466]
                  tunnel: w454 -> [w461]
                  tunnel: [w458] -> w449
                  stop <- w465 stop-if-true
                  (unwired) u32 620 ("identifier")
                  n165 = Unbundle By Name(w467) -> ("payload"=w462:u8[], "identifier"=w464:u32)
                  n166 = Equal?(x=w464, y=w466) -> (x = y?=w465:bool)
                  n167 = Index Array(array=w462) -> (element #1=w463:u8, element #2=w460:u8)  [unwired: 2 in]
                  n168 = case shown="Default" w464 {
                    selector: w464 -> [_ _ _ w522]
                    tunnel: w463 -> [w473 _ _ _]
                    tunnel: w460 -> [w472 _ _ _]
                    tunnel: w461 -> [w471 _ _ _]
                    tunnel: w462 -> [w470 w519 w521 w524]
                    tunnel: [w469 w519 w521 w524] -> w459
                    tunnel: [w468 "Read" "Read" w523] -> w458
                    frame 620 {
                      n169 = case shown="BF" w473 {
                        tunnel: w472 -> [w477 w488 _ _]
                        tunnel: w471 -> [_ w487 w515 _]
                        tunnel: w470 -> [w476 w486 _ w517]
                        tunnel: [w475 w485 w512 w517] -> w469
                        tunnel: [w474 w484 "Read" "Read"] -> w468
                        frame 111, Default {
                          n170 = case shown="2" w477 {
                            tunnel: w476 -> [w479 w481 w483]
                            tunnel: [w479 w481 w483] -> w475
                            tunnel: ["Read" "Read" "Read"] -> w474
                            frame 0, Default {
                            }
                            frame 1 {
                            }
                            frame 2 {
                            }
                          }
                        }
                        frame 98 {
                          n171 = case shown="6" w488 {
                            tunnel: w487 -> [_ w494 w500 w505 w510]
                            tunnel: w486 -> [w490 _ _ _ _]
                            tunnel: [w490 w492 w496 w502 w507] -> w485
                            tunnel: ["Read" "Read" "Read" "Read" "Read"] -> w484
                            frame 1, Default {
                            }
                            frame 4 {
                              # "GPS"
                              n172 = Unbundle By Name(w494) -> ("GPS"=w493:u8[][])
                              n173 = call "GPS_pcan.vi"("GPS data"=w493) -> ("GPS data 2"=w492:u8[])  [unwired: 10 in]
                            }
                            frame 3 {
                              n174 = Unbundle By Name(w500) -> ("macid"=w499:u8[])
                              n175 = Delete From Array(array=w499, length=2, index=0) -> (array with subset deleted=w496:u8[])  [unwired: 1 out]
                            }
                            frame 5 {
                              n176 = Unbundle By Name(w505) -> ("imei"=w504:u8[][])
                              n177 = call "Imei_PCAN.vi"("IMEI data"=w504) -> ("imei"=w503:string)  [unwired: 10 in]
                              n178 = String To Byte Array(string=w503) -> (unsigned byte array=w502:u8[])
                            }
                            frame 6 {
                              n179 = Unbundle By Name(w510) -> ("iccid"=w509:u8[][])
                              n180 = call "iccid_PCAN.vi"("iccid data"=w509) -> ("iccid"=w508:string)  [unwired: 10 in]
                              n181 = String To Byte Array(string=w508) -> (unsigned byte array=w507:u8[])
                            }
                          }
                        }
                        frame 99 {
                          n182 = Unbundle By Name(w515) -> ("Serial no."=w513:u8[][])
                          n183 = call "Barcode_decode.vi"("Barcode data"=w513) -> ("String 2"=w514:string)
                          n184 = String To Byte Array(string=w514) -> (unsigned byte array=w512:u8[])
                        }
                        frame 191 {
                        }
                      }
                    }
                    frame 623 {
                    }
                    frame 621 {
                    }
                    frame Default {
                      n185 = case shown="405, 707, 708, 729" w522 {
                        tunnel: ["Read" ("Message") "Error" ("Message")] -> w523
                        frame 1029, 1799, 1800, 1833 {
                        }
                        frame 1, Default {
                        }
                      }
                    }
                  }
                }
                n186 = Bundle By Name(cluster=w453, "ReadPayload"=w452, "String_Data"=w450) -> (w451:T8)
              }
            }
            "frame data" <- w427
          }
          frame True {
            n187 = call "Barcode_decode.vi"("Barcode data"=w531) -> ("String 2"=w529:string)
            n188 = String To Byte Array(string=w529) -> (unsigned byte array=w528:u8[])
            n189 = Bundle By Name(cluster=w533, "String_Data"=w532, "ReadPayload"=w528) -> (w534:T8)
          }
        }
        n190 = To Variant(anything=w395) -> (Variant=w404:variant)
        n191 = Bundle By Name(cluster=T6 {"Message"="", "Message Data"=variant} ("notification"), "Message"=w391, "Message Data"=w404) -> (w406:T6)
        n192 = Or(x=w410, y=w408) -> ()  [unwired: 1 out]
        n193 = Send Notification(notification=w406, notifier=w422) -> (notifier out=w405:refnum<notifier>)  [unwired: 1 in, 1 out]
        n194 = Bundle By Name(cluster=w396, "CAN_Read"=w402, "notifier out"=w405, "Repeatno."=u8 0, "P_queue"=w394) -> (w421:T7)
        n195 = call "Enque_Message_FGV.vi"("Priority"=TRUE, "error in (no error)"=w398, "Message"="Read", "queue IN"=w394) -> ("error out"=w397:errorcluster)  [unwired: 7 in]
      }
      frame "AddSignal" {
        # "Add Signal"
        n196 = Unbundle By Name(w556) -> ("P_queue"=w552:refnum<queue>, "CAN_MSGs_Write"=w555:T3)
        n197 = call "Add_Signal.vi"("CAN_MSGs"=w555) -> ("CAN_MSGs 2"=w553:T3)  [unwired: 10 in]
        n198 = Bundle By Name(cluster=w556, "CAN_MSGs_Write"=w553) -> (w554:T7)
        n199 = call "Enque_Message_FGV.vi"("error in (no error)"=w558, "Message Data"="Add Signal" ("\"Do Something Else\" button pressed"), "Message"="Update Display", "queue IN"=w552) -> ("error out"=w557:errorcluster)  [unwired: 7 in]
      }
      frame "DeleteSignal" {
        # "Delete Signal"
        n200 = Unbundle By Name(w565) -> ("CAN_MSGs_Write"=w564:T3, "P_queue"=w561:refnum<queue>)
        n201 = call "Delete_Signal.vi"("CAN_MSGs"=w564) -> ("CAN_MSGs 2"=w562:T3)  [unwired: 10 in]
        n202 = Bundle By Name(cluster=w565, "CAN_MSGs_Write"=w562) -> (w563:T7)
        n203 = call "Enque_Message_FGV.vi"("error in (no error)"=w567, "Message Data"="Delete Signal" ("\"Do Something Else\" button pressed"), "Message"="Update Display", "queue IN"=w561) -> ("error out"=w566:errorcluster)  [unwired: 7 in]
      }
      frame "Update Display" {
        # "Update Display - Convert the message data to a string to display in the Data Display indicator."
        n204 = Variant To Data(error in=w577, type="", Variant=w576) -> (data=→"Display <Replace Me>":string, error out=w574:errorcluster)
        n205 = Unbundle By Name(w572) -> ("CAN_MSGs_Write"=w571:T3)
        n206 = To Variant(anything=w571) -> (Variant=w570:variant)
        n207 = property on="CAN_MSGs" class="Clust"("Value"=w570) -> ()  [unwired: 2 in, 2 out]
        n208 = Merge Errors(w574) -> (w578:errorcluster)
      }
      frame "Uninit_PCAN" {
        n209 = Unbundle By Name(w583) -> ("Channel"=w580:u16)
        n210 = call <userlib>:"CAN Uninitialize.vi"("error in (no error)"=w582, "Channel"=w580) -> ("error out"=w581:errorcluster)  [unwired: 8 in, 1 out]
        n211 = call <vilib>:"Clear Errors.vi"("error in (no error)"=w581) -> ("error out"=w579:errorcluster)  [unwired: 5 in, 1 out]
      }
      frame "Error" {
        # "Error - Display an error dialog. This message is sent by the \"Error Handler\" VIs at the end of other loops in this application."
        n212 = Variant To Data(error in=w590, type=errorcluster {"status"=FALSE, "code"=0, "source"=""} ("error constant"), Variant=w589) -> (data=w587:errorcluster, error out=w586:errorcluster)
        n213 = call <vilib>:"Simple Error Handler.vi"("error in (no error)"=w587) -> ()  [unwired: 4 in, 5 out]
        n214 = disable-structure shown="Enabled" {
          disable-tunnel: w586 -> [w596 w597]
          disable-tunnel: [w593 w597] -> w585
          disable-tunnel: w584 -> [w592 _]
          frame Disabled {
            n215 = Unbundle By Name(w592) -> ("P_queue"=w591:refnum<queue>)
            n216 = Merge Errors(w596) -> (w594:errorcluster)
            n217 = call "Enque_Message_FGV.vi"("error in (no error)"=w594, "Message"="Initialize-PCAN", "queue IN"=w591) -> ("error out"=w593:errorcluster)  [unwired: 8 in]
          }
          frame Enabled {
          }
        }
      }
      frame "Confirm Quit" {
        # "Confirm Quit - Message that can confirm whether or not the user wants to exit the application."
        n218 = Unbundle By Name(w602) -> ("P_queue"=w601:refnum<queue>, "Channel"=w600:u16)
        n219 = call <userlib>:"CAN Uninitialize.vi"("error in (no error)"=w599, "Channel"=w600) -> ("error out"=w598:errorcluster)  [unwired: 8 in, 1 out]
        n220 = call "Enque_Message_FGV.vi"("Priority"=TRUE ("Priority Message? (F)"), "error in (no error)"=w598, "Message"="Exit", "queue IN"=w601) -> ("error out"=w605:errorcluster)  [unwired: 7 in]
        n221 = Merge Errors(w605) -> (w606:errorcluster)
      }
      frame "Exit" {
        # "Stop the VI"
        # "Release the message queue reference"
        # "Exit - Exit the application."
        n222 = Unbundle By Name(w614) -> ("notifier out"=w613:refnum<notifier>, "Channel"=w607:u16, "P_queue"=w611:refnum<queue>)
        n223 = Release Notifier(notifier=w613, error in (no error)=w609) -> (error out=w612:errorcluster)  [unwired: 1 in, 2 out]
        n224 = call "Queue_Comm_FGV.vi"("error in (no error)"=w609, "Enum"=FGV_Queue_Control."Release", "queue in"=w611) -> ("error Out"=w618:errorcluster)  [unwired: 7 in, 1 out]
        n225 = call "Fire User Event - Stop.vi"("User Event - Stop"=w617) -> ("error out"=w615:errorcluster)  [unwired: 10 in]
        n226 = call "Fire User Event - Stop.vi"("User Event - Stop"=w620) -> ("error out"=w616:errorcluster)  [unwired: 10 in]
        n227 = Merge Errors(w612, w616, w615, w618) -> (w621:errorcluster)
        n228 = call <vilib>:"Clear Errors.vi"("error in (no error)"=w621) -> ("error out"=w610:errorcluster)  [unwired: 5 in, 1 out]
        n229 = call <userlib>:"CAN Uninitialize.vi"("error in (no error)"=w610, "Channel"=w607) -> ("error out"=w608:errorcluster)  [unwired: 8 in, 1 out]
      }
      frame Default {
        # "'Default' case only runs if there is a message that isn't defined in any of the other cases.  Output a programming error."
        n230 = xnode "Error Ring"("parameter 0"=w624) -> ("error out"=w623:errorcluster)
        n231 = call <vilib>:"Simple Error Handler.vi"("error in (no error)"=w623) -> ()  [unwired: 4 in, 5 out]
      }
    }
    n232 = call "Error_Handler_MHL_FGV.vi"("Case"=w32, "error in (no error)"=w41, "VI_name"=w33, "queue IN"=w34) -> ("error Out"=w40:errorcluster)  [unwired: 7 in]
  }
  n233 = while {
    shift-right: [w637] -> w25
    shift-left: w22 -> [w638]
    tunnel: [w634] -> w23
    tunnel: w9 -> [w633]
    stop <- w636 stop-if-true
    # "Event Handling Loop"
    n234 = event shown="[7] \"Exit\": Value Change" {
      selector: w638 -> [_ _ _ _ _ _ _ _ _]
      dyn-events: [_ _ _ _ _ _ _ _ _] -> w637
      timeout: _ -> [_ _ _ _ _ _ _ _ _]
      tunnel: [_ _ _ _ _ _ _ _ TRUE ("Discard?")] -> w636
      tunnel: [w641 w644 w650 w654 w658 w664 _ w669 _] -> w635
      tunnel: w633 -> [w639 w643 w647 w653 w657 w661 _ w666 _]
      event "Write_PCAN": Value Change {
        n235 = event-data() -> ()  [unwired: 1 in, 1 out]
        n236 = call "Enque_Message_FGV.vi"("Priority"=TRUE ("Priority Message? (F)"), "Message"="Write", "queue IN"=w639) -> ("error out"=w641:errorcluster)  [unwired: 8 in]
      }
      event Value Change {
        n237 = event-data() -> ()  [unwired: 1 in, 1 out]
        n238 = call "Enque_Message_FGV.vi"("Priority"=TRUE ("Priority Message? (F)"), "Message"="AddSignal", "queue IN"=w643) -> ("error out"=w644:errorcluster)  [unwired: 8 in]
      }
      event Value Change {
        n239 = event-data() -> ()  [unwired: 1 in, 1 out]
        n240 = To Variant(anything="CAN_MSGs") -> (Variant=w648:variant)
        n241 = call "Enque_Message_FGV.vi"("Priority"=TRUE ("Priority Message? (F)"), "Message Data"=w648, "Message"="FrameSignal", "queue IN"=w647) -> ("error out"=w650:errorcluster)  [unwired: 7 in]
      }
      event Value Change {
        n242 = event-data() -> ()  [unwired: 1 in, 1 out]
        n243 = call "Enque_Message_FGV.vi"("Priority"=TRUE ("Priority Message? (F)"), "Message"="DeleteSignal", "queue IN"=w653) -> ("error out"=w654:errorcluster)  [unwired: 8 in]
      }
      event "Read_PCAN": Value Change {
        n244 = event-data() -> ()  [unwired: 1 in, 1 out]
        n245 = call "Enque_Message_FGV.vi"("Priority"=TRUE ("Priority Message? (F)"), "Message"="ConfigRead", "queue IN"=w657) -> ("error out"=w658:errorcluster)  [unwired: 8 in]
      }
      event Panel Close? {
        n246 = event-data() -> ()  [unwired: 1 in, 1 out]
        n247 = call "Enque_Message_FGV.vi"("Priority"=TRUE ("Priority Message? (F)"), "Message"="Confirm Quit", "queue IN"=w661) -> ("error out"=w664:errorcluster)  [unwired: 8 in]
        n248 = event-data("Discard?"=TRUE) -> ()  [unwired: 1 in, 1 out]
      }
      event Application Instance Close {
        # "#CodeRecommended - When a project closes, all VIs within that project are aborted and leave memory. However, any code placed in this event frame is guaranteed to run to completion, so add any cleanup code that absolutely must happen here."
        n249 = event-data() -> ()  [unwired: 1 in, 1 out]
      }
      event "Exit": Value Change {
        n250 = event-data() -> ()  [unwired: 1 in, 1 out]
        n251 = call "Enque_Message_FGV.vi"("Priority"=TRUE ("Priority Message? (F)"), "Message"="Confirm Quit", "queue IN"=w666) -> ("error out"=w669:errorcluster)  [unwired: 8 in]
      }
      event User Event {
        n252 = event-data() -> ()  [unwired: 1 in, 1 out]
        n253 = local write "Display <Replace Me>"("\"Exit\" button pressed" ("VI Stopped")) -> ()
      }
    }
    n254 = call "Error_Handler_EHL_FGV.vi"("error in (no error)"=w635, "queue IN"=w633) -> ("error Out"=w634:errorcluster)  [unwired: 9 in]
  }
  n255 = Unregister For Events(event registration refnum=w25, error in=w23) -> (error out=w26:errorcluster)
  n256 = Merge Errors(w26, w29) -> (w27:errorcluster)
  n257 = call "Destroy User Event - Stop.vi"("error in (no error)"=w27, "User Event - Stop"=w11) -> ("error out"=→"error in (out)":errorcluster)  [unwired: 9 in]
